vi "TWM Measure.vi"(0 "handle":i32, 1 "end of packet key":string="TWM:command:EndOfPacket", 3 "timeout [s] (10s)":dbl=30.0, 5 "meas root path (last)":path, 7 "quantity names (all)":string[](array[string]), 9 "stop ref (none)":refnum<vi>, 11 "error in":errorcluster, 12 "qwtb maxdim (scalar)":T3 caption="Max. shown dimension (scalar)", 13 "status ref (none)":refnum<vi>, 14 "phase ref channel tag (none)":string) -> (4 "handle out":i32, 6 "data":T2[][](array[typedef]), 8 "stoped?":bool, 10 "quantities":T1, 15 "error out":errorcluster)   [LabVIEW 2020]
doc: "TWM client top level function: Start measurement, wait for completion, Get result.\n\nSet reasonable timeout for the TWM sampling and processing. Wire in the the 'stop' reference to allow termination of the TWM task."
uses:
  external libraries/TWM client.lvlibp/server/TWM client/TWM Client Result Max Dim.ctl
  external libraries/TWM client.lvlibp/server/TWM client/TWM Client Quantity Record.ctl
  external libraries/TWM client.lvlibp/server/TWM client/TWM Client Result Info.ctl
  <vilib>/ErrorRing/Error Ring.xnode
  external libraries/TWM client.lvlibp
  <vilib>/Utility/error.llb/Error Cluster From Error Code.vi
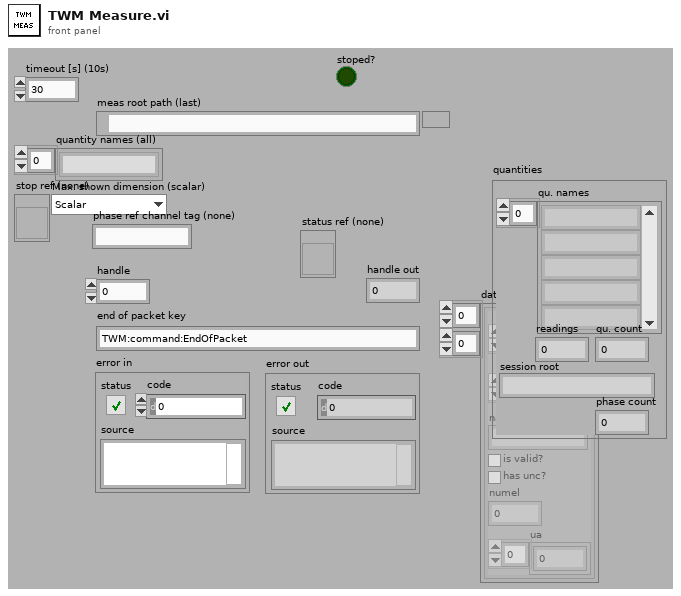
[diagram p1: front panel]
types:
  T1 = typedef "TWM client.lvlibp/TWM Client Result Info.ctl" = cluster{"qu. names":string[], "readings":i32, "qu. count":i32, "session root":string, "phase count":i32}
  T2 = typedef "TWM client.lvlibp/TWM Client Quantity Record.ctl" = cluster{"val":dbl[], "unc":dbl[], "name":string, "is valid?":bool, "has unc?":bool, "numel":i32, "ua":dbl[]}
  T3 = typedef "TWM client.lvlibp/TWM Client Result Max Dim.ctl" = enum16{"Scalar", "Vector", "Matrix"}
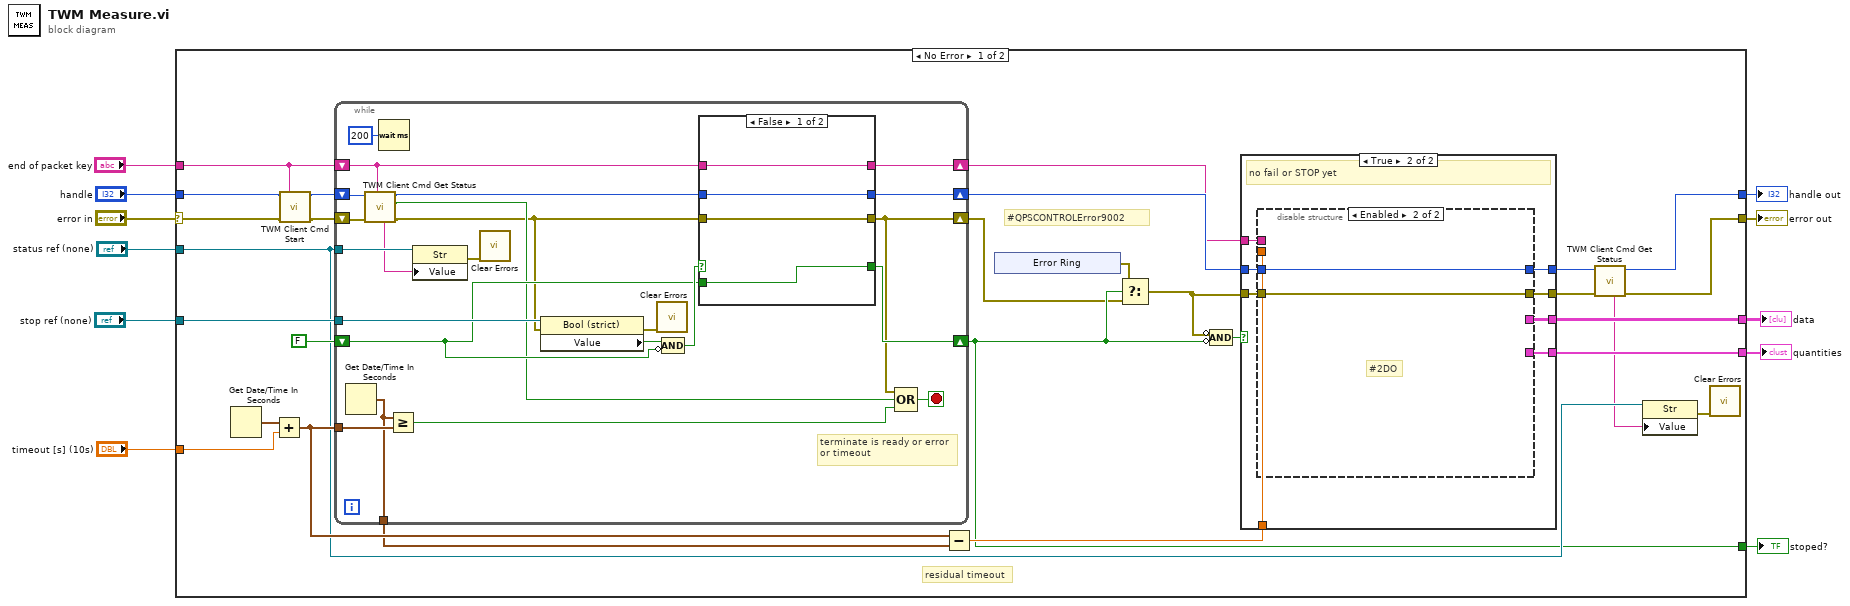
[diagram p0: block diagram]
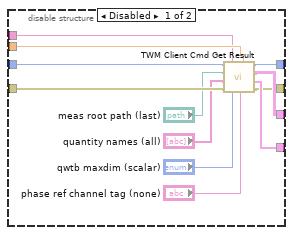
[diagram p3: hidden frame]
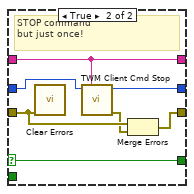
[diagram p4: hidden frame]
diagram:
  n1 = case shown="No Error" "error in" {
    selector: "error in" -> [w26 w104]
    tunnel: "handle" -> [w27 w103]
    tunnel: "stop ref (none)" -> [w39 _]
    tunnel: "timeout [s] (10s)" -> [w37 _]
    tunnel: "end of packet key" -> [w23 _]
    tunnel: [w21 w103] -> w7
    tunnel: [w19 w104] -> w6
    tunnel: [w29 _] -> w5
    tunnel: [w28 _] -> w4
    tunnel: [w15 _] -> w2
    tunnel: "status ref (none)" -> [w17 _]
    frame No Error {
      # "#QPSCONTROLError9002"
      # "residual timeout"
      n2 = Get Date/Time In Seconds() -> (seconds since 1Jan1904=w36:timestamp)
      n3 = Add(x=w36, y=w37) -> (x+y=w35:timestamp)
      n4 = call "TWM Client Cmd Start.vi"("end of packet key"=w23, "error in"=w26, "handle"=w27) -> ("error out"=w25:errorcluster, "handle out"=w24:i32)  [unwired: 7 in]
      n5 = while {
        shift-right: [w89] -> w32
        shift-left: w24 -> [w73]
        shift-right: [w83] -> w13
        shift-left: w25 -> [w74]
        tunnel: w39 -> [w90]
        shift-right: [w88] -> w15
        shift-left: FALSE -> [w85]
        tunnel: w35 -> [w84]
        tunnel: [w79] -> w34
        shift-right: [w78] -> w30
        shift-left: w23 -> [w72]
        tunnel: w17 -> [w71]
        stop <- w81 stop-if-true
        # "terminate is ready or error\nor timeout"
        n6 = Get Date/Time In Seconds() -> (seconds since 1Jan1904=w79:timestamp)
        n7 = call "TWM Client Cmd Get Status.vi"("end of packet key"=w72, "error in"=w74, "handle"=w73) -> ("error out"=w75:errorcluster, "ready?"=w76:bool, "handle out"=w77:i32, "status string"=w70:string)  [unwired: 4 in, 1 out]
        n8 = Wait (ms)(milliseconds to wait=u32 200) -> ()  [unwired: 1 out]
        n9 = Greater Or Equal?(x=w79, y=w84) -> (x >= y?=w82:bool)
        n10 = property class="Str"(reference=w71, "Value"=w70) -> (error out=w69:errorcluster)  [unwired: 1 in, 1 out]
        n11 = call <vilib>:"Clear Errors.vi"("error in (no error)"=w69) -> ()  [unwired: 5 in, 2 out]
        n12 = property class="Bool (strict)"(reference=w90, error in=w75) -> (error out=w91:errorcluster, "Value"=w87:bool)  [unwired: 1 out]
        n13 = call <vilib>:"Clear Errors.vi"("error in (no error)"=w91) -> ()  [unwired: 5 in, 2 out]
        n14 = Compound Arithmetic op=AND(w87, invert w85) -> (w86:bool)
        n15 = case shown="False" w86 {
          selector: w86 -> [_ w100]
          tunnel: w75 -> [w95 w102]
          tunnel: w77 -> [w94 w97]
          tunnel: [w94 w99] -> w89
          tunnel: [w95 w101] -> w83
          tunnel: [w93 w100] -> w88
          tunnel: w85 -> [w93 _]
          tunnel: w72 -> [w92 w98]
          tunnel: [w92 w98] -> w78
          frame False {
          }
          frame True {
            # "STOP command\nbut just once!"
            n16 = call <vilib>:"Clear Errors.vi"("error in (no error)"=w102) -> ()  [unwired: 5 in, 2 out]
            n17 = call "TWM Client Cmd Stop.vi"("end of packet key"=w98, "handle"=w97) -> ("error out"=w96:errorcluster, "handle out"=w99:i32)  [unwired: 8 in]
            n18 = Merge Errors(w102, w96) -> (w101:errorcluster)
          }
        }
        n19 = Compound Arithmetic op=OR(w83, w76, w82) -> (w81:bool)
      }
      n20 = Subtract(x=w35, y=w34) -> (x-y=w31:dbl)
      n21 = xnode "Error Ring"() -> ("error out"=w12:errorcluster)
      n22 = Select(t=w12, s=w15, f=w13) -> (s? t:f=w14:errorcluster)
      n23 = Compound Arithmetic op=AND(invert w14, invert w15) -> (w33:bool)
      n24 = case shown="True" w33 {
        tunnel: w14 -> [w46 w49]
        tunnel: w32 -> [w45 w54]
        tunnel: [w46 w50] -> w20
        tunnel: [w45 w53] -> w22
        tunnel: w31 -> [_ w48]
        tunnel: w30 -> [_ w47]
        tunnel: [_ w52] -> w29
        tunnel: [_ w51] -> w28
        frame False {
          # "STOP or error"
        }
        frame True {
          # "no fail or STOP yet"
          n25 = disable-structure shown="Enabled" {
            disable-tunnel: w54 -> [w66 w67]
            disable-tunnel: [w65 w67] -> w53
            disable-tunnel: [w64 _] -> w52
            disable-tunnel: [w63 _] -> w51
            disable-tunnel: [w62 w68] -> w50
            disable-tunnel: w49 -> [w61 w68]
            disable-tunnel: w48 -> [w56 _]
            disable-tunnel: w47 -> [w55 _]
            frame Disabled {
              n26 = call "TWM Client Cmd Get Result.vi"("phase ref channel tag (none)"="phase ref channel tag (none)", "timeout [s] (10s)"=w56, "qwtb maxdim (scalar)"="qwtb maxdim (scalar)", "end of packet key"=w55, "error in"=w61, "quantity names (all)"="quantity names (all)", "meas root path (last)"="meas root path (last)", "handle"=w66) -> ("error out"=w62:errorcluster, "result info"=w63:T1, "result data"=w64:T2[][], "handle out"=w65:i32)
            }
            frame Enabled {
              # "#2DO"
            }
          }
        }
      }
      n27 = call "TWM Client Cmd Get Status.vi"("error in"=w20, "handle"=w22) -> ("error out"=w19:errorcluster, "handle out"=w21:i32, "status string"=w16:string)  [unwired: 5 in, 2 out]
      n28 = property class="Str"(reference=w17, "Value"=w16) -> (error out=w18:errorcluster)  [unwired: 1 in, 1 out]
      n29 = call <vilib>:"Clear Errors.vi"("error in (no error)"=w18) -> ()  [unwired: 5 in, 2 out]
    }
    frame Error {
    }
  }
  "error out" <- w6
  "handle out" <- w7
  "data" <- w5
  "quantities" <- w4
  "stoped?" <- w2
